vi "WPI_UtilitiesFRC Build Error.vi"(0 "error code":i32, 5 "extra error text":string, 7 "chain levels to remove (1)":i32=1, 9 "include timestamp? (T)":bool=TRUE, 11 "error in (no error)":errorcluster) -> (15 "error out":errorcluster)   [LabVIEW 2025]
uses:
  <vilib>/Utility/error.llb/whitespace.ctl
  <vilib>/Utility/error.llb/Trim Whitespace One-Sided.vi
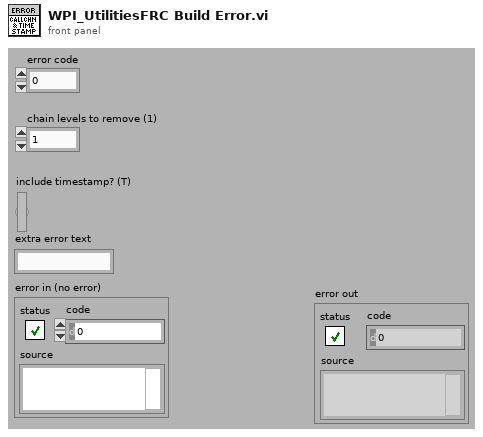
[diagram p1: front panel]
types:
  T1 = typedef "whitespace.ctl" = u16
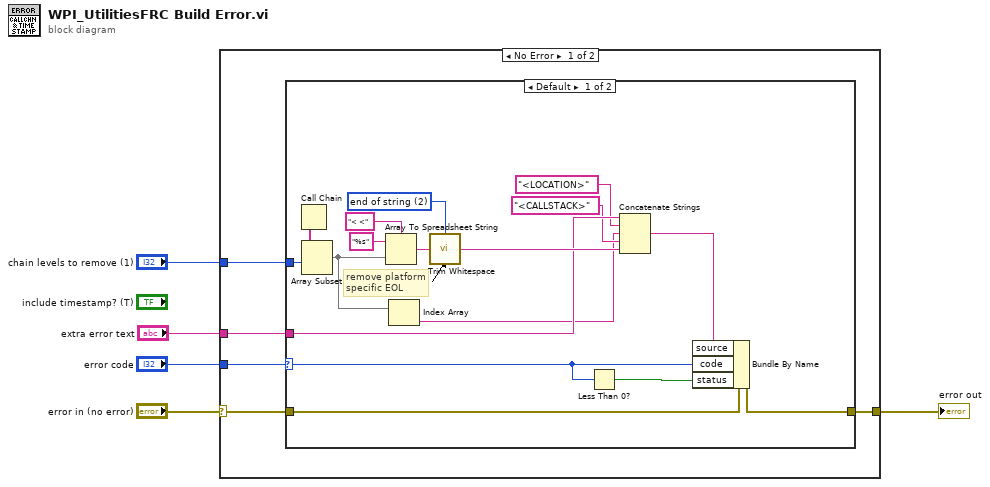
[diagram p0: block diagram]
diagram:
  n1 = case shown="No Error" "error in (no error)" {
    selector: "error in (no error)" -> [w9 w29]
    tunnel: "chain levels to remove (1)" -> [w10 _]
    tunnel: [w7 w29] -> w3
    tunnel: "error code" -> [w8 _]
    tunnel: "extra error text" -> [w6 _]
    frame No Error {
      n2 = case shown="Default" w8 {
        selector: w8 -> [w18 _]
        tunnel: w10 -> [w25 _]
        tunnel: w9 -> [w17 w28]
        tunnel: [w16 w28] -> w7
        tunnel: w6 -> [w15 _]
        frame Default {
          w19 = T1 2 items=["both", "start of string", "end of string"] ("location (both)")
          # "remove platform specific EOL"
          n3 = Call Chain() -> (call chain=w24:string[])
          n4 = Array Subset(array=w24, index=w25) -> (w12:string[])  [unwired: 1 in]
          n5 = Array To Spreadsheet String(delimiter (Tab)="< <", array=w12, 3:"%s" ("format string")) -> (spreadsheet string=w21:string)
          n6 = Index Array(array=w12) -> (element=w11:string)  [unwired: 1 in]
          n7 = call <vilib>:"Trim Whitespace.vi"("string"=w21, "location (both)"=w19) -> ("trimmed string"=w22:string)
          n8 = Less Than 0?(x=w18) -> (x < 0?=w23:bool)
          n9 = Concatenate Strings(w15, "<LOCATION>" ("string"), w11, "<CALLSTACK>" ("string"), w22) -> (w20:string)
          n10 = Bundle By Name(cluster=w17, "source"=w20, "code"=w18, "status"=w23) -> (w16:errorcluster)
        }
        frame 0 {
        }
      }
    }
    frame Error {
    }
  }
  "error out" <- w3
